vi "ROI to Rect.vi"(8 "error in (no error)":errorcluster, 11 "ROI":T1) -> (0 "error out":errorcluster, 3 "Rect":i32[](array[numeric]))   [LabVIEW 2023]
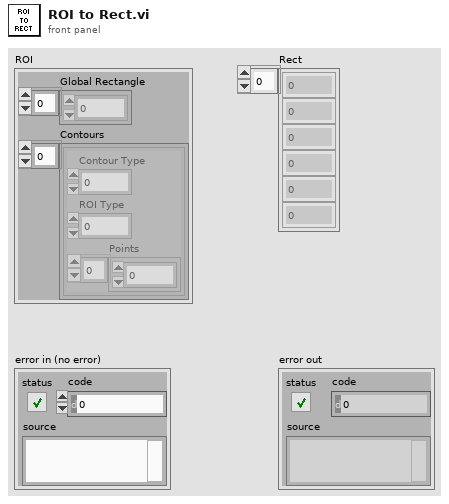
[diagram p1: front panel]
types:
  T1 = cluster{"Global Rectangle":i32[], "Contours":cluster{"Contour Type":u32, "ROI Type":u32, "Points":i32[]}[]}
  T2 = typedef "IMAQ Rectangle" = cluster{"Left":i32, "Top":i32, "Right":i32, "Bottom":i32, "Rotation":dbl}
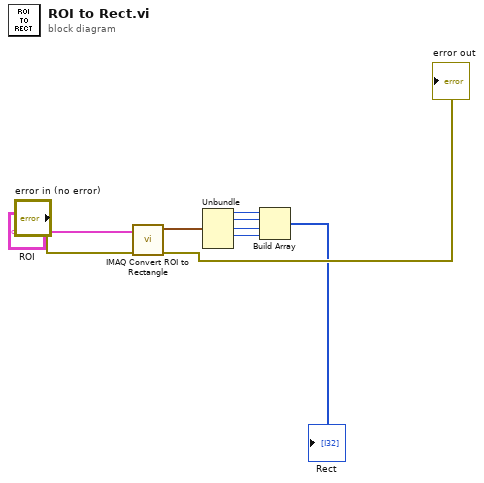
[diagram p0: block diagram]
diagram:
  n1 = call "IMAQ Convert ROI to Rectangle"("error in (no error)"="error in (no error)", "ROI Descriptor"="ROI") -> ("error out"=→"error out":errorcluster, "Rectangle"=w1:T2)  [unwired: 7 in]
  n2 = Unbundle(w1) -> ("Left"=w2:i32, "Top"=w3:i32, "Right"=w4:i32, "Bottom"=w5:i32)  [unwired: 1 out]
  n3 = Build Array(w2, w3, w4, w5) -> (→"Rect":i32[])
